vi "Create All Message Queues.vi"(8 "error in (no error)":errorcluster, 11 "Data":T1={"offset"=99.0, "time"=""} {"offset" format="%.3g"}) -> (0 "error out":errorcluster, 3 "Message Queues out":T2)   [LabVIEW 2018, in "Message Queue.lvlib"]
doc: "This VI creates and initializes all the message queues for your application. If your application requires more than one message queue, right-click the \"Message Queues\" constant above and select Open Type Def. Add the new Message Queue(s) to the type definition, then initialize them in this VI."
uses:
  Message Queue.lvlib
  All Message Queues.ctl
  Message Cluster.ctl
  Controls/Data Queue.ctl
  Controls/Acquired Data.ctl
  Controls/Data Notifier.ctl
  Enqueue Message (Single).vi
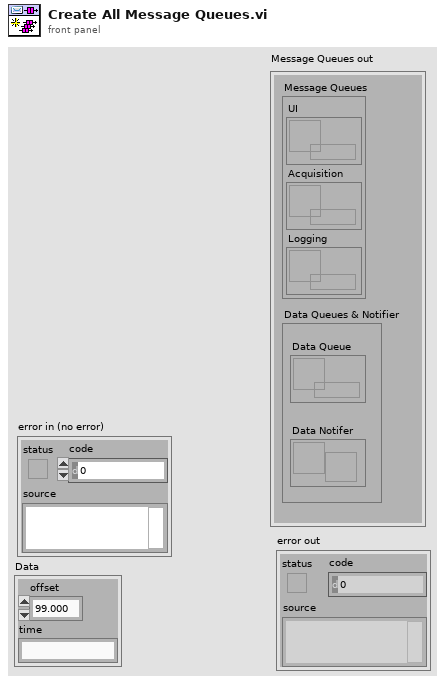
[diagram p1: front panel]
types:
  T1 = typedef "Acquired Data.ctl" = cluster{"offset":dbl, "time":string}
  T2 = typedef "Message Queue.lvlib/All Message Queues.ctl" = cluster{"Message Queues":cluster{"UI":refnum<queue>, "Acquisition":refnum<queue>, "Logging":refnum<queue>}, "Data Queues & Notifier":cluster{"Data Queue":T3, "Data Notifer":T4}}
  T3 = typedef "Data Queue.ctl" = refnum<queue>
  T4 = typedef "Data Notifier.ctl" = refnum<notifier>
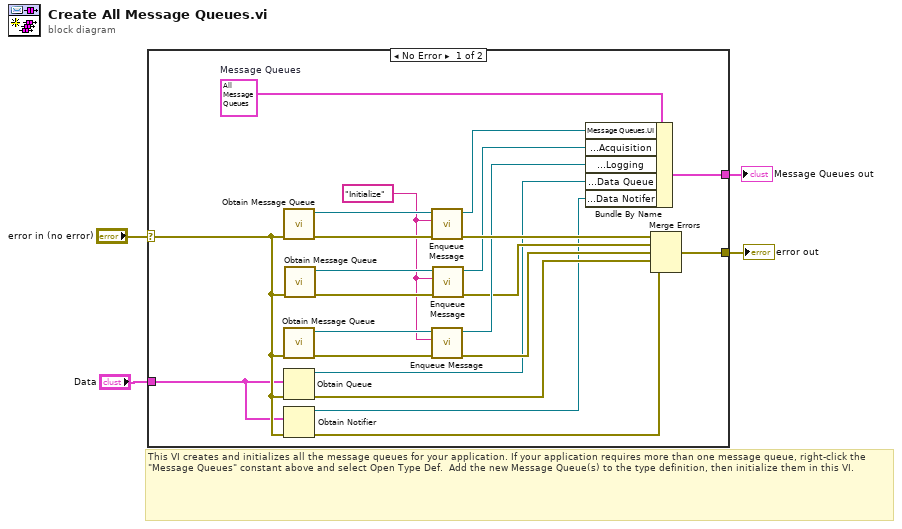
[diagram p0: block diagram]
diagram:
  # "This VI creates and initializes all the message queues for your application. If your application requires more than one message queue, right-click the \"Message Queues\" constant above and select Open Type Def.  Add the new Message Queue(s) to the type definition, then initialize them in this VI."
  n1 = case shown="No Error" "error in (no error)" {
    selector: "error in (no error)" -> [w10 w27]
    tunnel: [w13 w27] -> w4
    tunnel: [w24 _] -> w3
    tunnel: "Data" -> [w9 _]
    frame No Error {
      w17 = "Initialize" ("Message")
      w25 = T2 {"Message Queues"={"UI"=refnum, "Acquisition"=refnum, "Logging"=refnum}, "Data Queues & Notifier"={"Data Queue"=refnum, "Data Notifer"=refnum}}  # Message Queues
      n2 = call "Obtain Message Queue.vi"("error in (no error)"=w10) -> ("error out"=w23:errorcluster, "Message Queue"=w22:refnum<queue>)  [unwired: 9 in]
      n3 = call "Obtain Message Queue.vi"("error in (no error)"=w10) -> ("error out"=w19:errorcluster, "Message Queue"=w18:refnum<queue>)  [unwired: 9 in]
      n4 = Obtain Queue(element data type=w9, error in (no error)=w10) -> (queue out=w6:refnum<queue>, error out=w8:errorcluster)  [unwired: 3 in, 1 out]
      n5 = Obtain Notifier(notification data type=w9, error in (no error)=w10) -> (notifier out=w5:refnum<notifier>, error out=w7:errorcluster)  [unwired: 2 in, 1 out]
      n6 = call "Obtain Message Queue.vi"("error in (no error)"=w10) -> ("error out"=w20:errorcluster, "Message Queue"=w21:refnum<queue>)  [unwired: 9 in]
      n7 = call-poly "Enqueue Message.vi"("error in (no error)"=w23, "Message"=w17, "Message Queue"=w22) -> ("error out"=w26:errorcluster, "dup Message Queue"=w16:refnum<queue>)  [unwired: 7 in]
      n8 = call-poly "Enqueue Message.vi"("error in (no error)"=w19, "Message"=w17, "Message Queue"=w18) -> ("error out"=w11:errorcluster, "dup Message Queue"=w14:refnum<queue>)  [unwired: 7 in]
      n9 = call-poly "Enqueue Message.vi"("error in (no error)"=w20, "Message"=w17, "Message Queue"=w21) -> ("error out"=w12:errorcluster, "dup Message Queue"=w15:refnum<queue>)  [unwired: 7 in]
      n10 = Bundle By Name(cluster=w25, "Message Queues.UI"=w16, "Message Queues.Acquisition"=w15, "Message Queues.Logging"=w14, "Data Queues & Notifier.Data Queue"=w6, "Data Queues & Notifier.Data Notifer"=w5) -> (w24:T2)
      n11 = Merge Errors(w26, w12, w11, w8, w7) -> (w13:errorcluster)
    }
    frame Error {
    }
  }
  "Message Queues out" <- w3
  "error out" <- w4
